vi "Pure Pursuit.vi"(0 "Lookahead":dbl, 1 "Trackwidth":dbl=30.0 format="%#_13g", 2 "kffv":dbl, 3 "kffa":dbl, 5 "Odometry":T1, 7 "Max Velocity":dbl, 9 "Max Accel":dbl, 11 "error in (no error)":errorcluster) -> (4 "Left Velocity":dbl, 6 "Right Velocity":dbl, 8 "Target Point":T2, 10 "Close Point":T2, 12 "Finished?":bool, 13 "index out":i32, 14 "Curvature":dbl, 15 "error out":errorcluster)   [LabVIEW 2018, in "Pure Pursuit.lvlib"]
uses:
  Pure Pursuit.lvlib
  Typedef/Path Point.ctl
  Odometry/Typedef/Odometry.ctl
  Odometry/Typedef/Velocity Data.ctl
panel:
  in  "Min Velocity":dbl=25.0
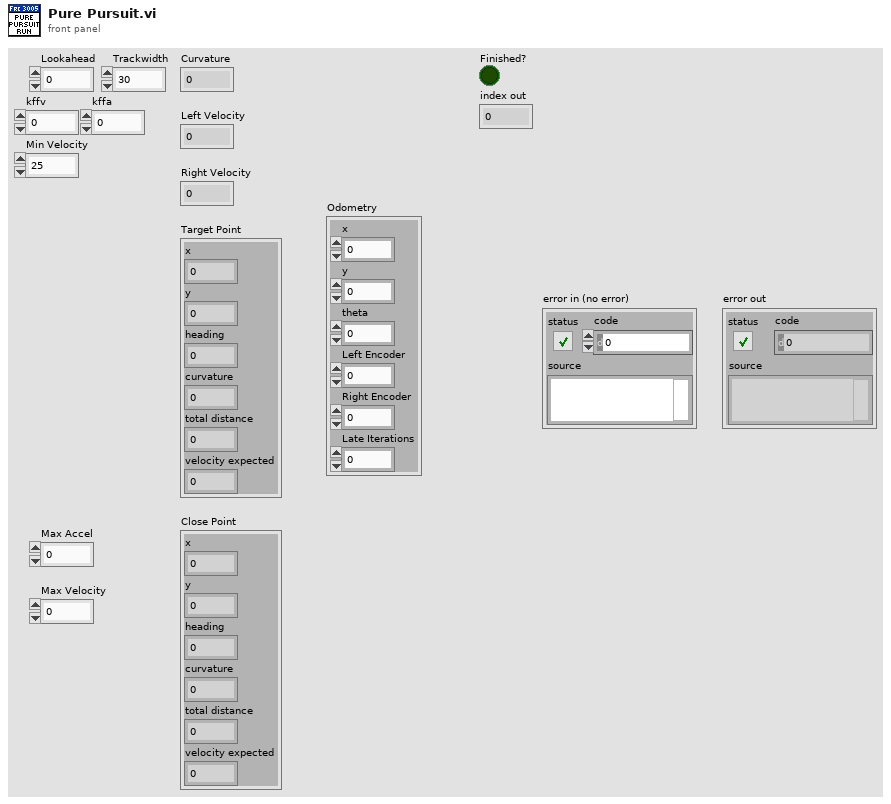
[diagram p1: front panel]
types:
  T1 = typedef "Odometry.ctl" = cluster{"x":dbl, "y":dbl, "theta":dbl, "Left Encoder":dbl, "Right Encoder":dbl, "Late Iterations":i16}
  T2 = typedef "Pure Pursuit.lvlib/Path Point.ctl" = cluster{"x":dbl, "y":dbl, "heading":dbl, "curvature":dbl, "total distance":dbl, "velocity expected":dbl}
  T3 = typedef "Velocity Data.ctl" = cluster{"Right Velocity Raw":sgl, "Left Velocity Raw":sgl}
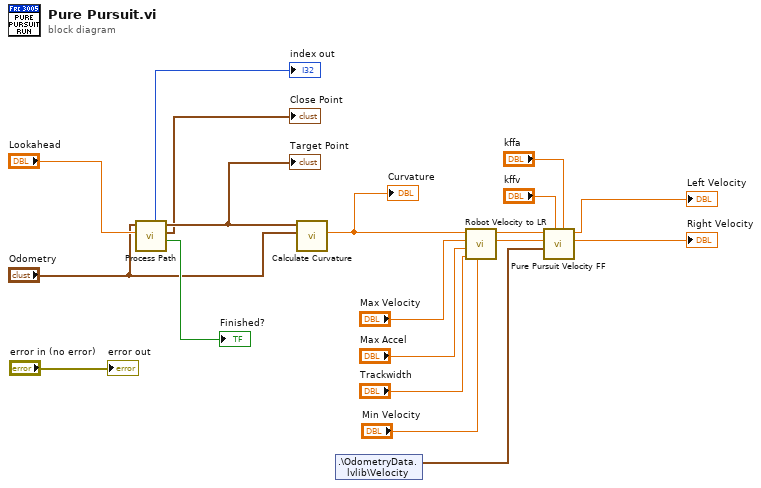
[diagram p0: block diagram]
diagram:
  n1 = call "Process Path.vi"("Lookahead"="Lookahead", "Odometry"="Odometry") -> ("Finished?"=→"Finished?":bool, "Close Point"=→"Close Point":T2, "Target Point"=w18:T2, "index out"=→"index out":i32)  [unwired: 6 in]
  "Target Point" <- w18
  n2 = call "Calculate Curvature.vi"("Odometry"="Odometry", "Target Point"=w18) -> ("Curvature"=w17:dbl)  [unwired: 8 in, 1 out]
  "Curvature" <- w17
  n3 = shared-variable ".\\OdometryData.lvlib\\Velocity"() -> (w2:T3)  [unwired: 1 in, 1 out]
  n4 = call "Robot Velocity to LR.vi"("Min Velocity"="Min Velocity", "Trackwidth"="Trackwidth", "Max Accel"="Max Accel", "Max Velocity"="Max Velocity", "Curvature"=w17) -> ("r"=w9:dbl, "l"=w10:dbl)  [unwired: 5 in]
  n5 = call "Pure Pursuit Velocity FF.vi"("kffa"="kffa", "kffv"="kffv", "Velocity"=w2, "Right Desired Velocity"=w9, "Left Desired Velocity"=w10) -> ("Right Velocity"=→"Right Velocity":dbl, "Left Velocity"=→"Left Velocity":dbl)  [unwired: 5 in]
  "error out" <- "error in (no error)"
